vi "Generate LabVIEW FPGA Code for Exponentially Weighted Moving Average Filter.vi"() -> ()   [LabVIEW 2023]
doc: "Demonstrates how to use the Digital Filter Design VIs to design, analyze, and generate LabVIEW FPGA code from a fixed-point, exponentially weighted moving average filter.\n\nComplete the following steps to use this VI.\n1) Specify a valid <B>Destination Folder</B> for code generation.\n2) Specify a <B>Filter Name</B> for code generation.\n3) Specify the number of channels that you want the filter to process in the <B># Channels</B> input.\n4) Run the VI. The <B>Maximum Input Fs@40 MHz FPGA Clock</B> output returns a value that indicates the processing power of the generated filter block."
uses:
  <vilib>/addons/Digital Filter Design/FXPModel.llb/DFD FXP Quantize Coef (Easy).vi
  <vilib>/addons/Digital Filter Design/Analysis.llb/DFD Plot Freq Response (Linear-Spaced).vi
  <vilib>/addons/Digital Filter Design/CodeGen.llb/DFD FXP LabVIEW FPGA Code Generator.vi
  <vilib>/addons/Digital Filter Design/NI_DigFilterLicensed.lvlib
panel:
  out "Magnitude Response":cluster{"f0":dbl, "df":dbl, "values":dbl[]}[](graph)
  in  "Coefficients b/v Word Length":i16=16
  in  "Coefficients a/k Word Length":i16=16
  in  "Sampling Frequency [Hz]":dbl=1000.0 format="%0.2f"
  in  "Time Constant [s]":dbl=0.1 format="%.2f"
  in  "Gain Settings":T1={"gain processing"=1, "gain word length"=16} {"gain processing" items=["On Target", "On Host"]}
  out "Maximum Input Fs@40 MHz FPGA Clock":dbl format="%#_5p Hz"
  out "lvproj Path":path
  in  "Open Project?":bool=TRUE
  in  "Filter Name":string
  in  "# Channels":i32=1
  in  "Destination Folder":path
  in  "Output Word Length":i16=16
  in  "Input Word Length":i16=16
  out "Error Message":string
  # "Select Help>>Show Context Help and move the cursor over the VI icon for more information."
  # "Filter Settings"
  # "Modeling Settings"
  # "Code Generation Settings"
  # "Code Generation Feedback"
  # "Quantization Settings"
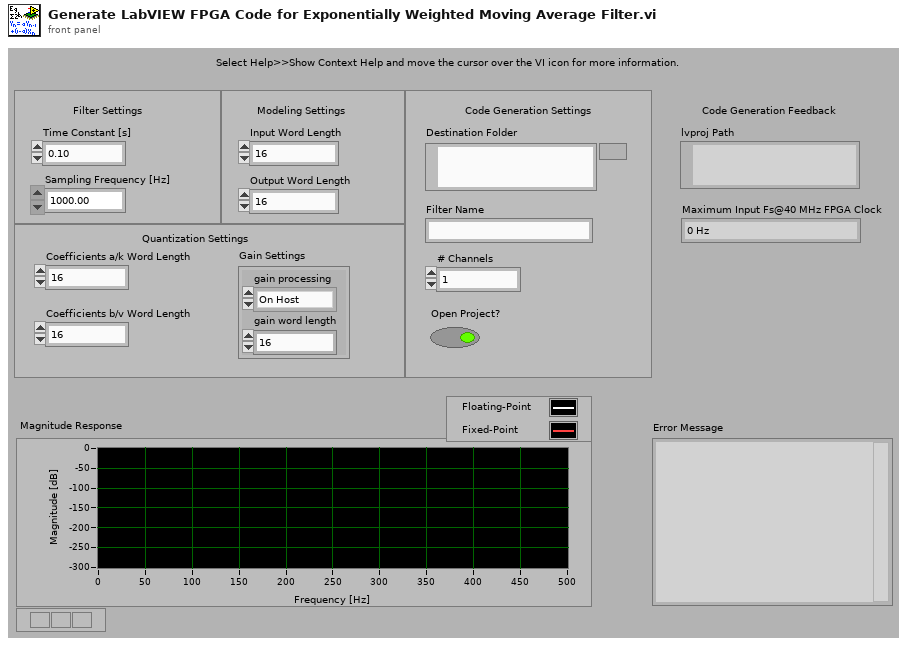
[diagram p1: front panel]
types:
  T1 = cluster{"gain processing":u16, "gain word length":i16}
  T2 = typedef "NI_DigFilterLicensed.lvlib/DFD Filter Obj.ctl" = cluster{"mSRate_Fs":dbl, "mSRate_Version":string, "mSRate_Comments":string, "mSRate_OrgCoef":T3, "mSRate_CurCoef":T3, "mSRate_Quantized?":bool, "mSRate_QCoef":T3, "mSRate_QSettings":T5[], "mSRate_Order":i32, "mSRate_Scaling":cluster{"mSRate_ScaleByPowerOf2?":bool, "mSRate_ScaleType":T7}}
  T3 = typedef "NI_DigFilterLicensed.lvlib/DFD Filter Coef.ctl" = cluster{"type":T4, "gain":dbl, "coef a (k)":dbl[], "coef b (v)":dbl[]}
  T4 = typedef "NI_DigFilterLicensed.lvlib/DFD Filter Structure Type Selector.ctl" = enum16{"Undefined", "FIR Direct Form", "FIR Direct Form Transposed", "FIR Symmetric", "FIR Antisymmetric", "IIR Direct Form I", "IIR Direct Form I Transposed", "IIR Direct Form II", "IIR Direct Form II Transposed", "IIR Cascaded Second Order Sections Form I", "IIR Cascaded Second Order Sections Form I Transposed", "IIR Cascaded Second Order Sections Form II", "IIR Cascaded Second Order Sections Form II Transposed", "Lattice Allpass (basic sections)", "Lattice Allpass (one multiplier sections)", "Lattice Allpass (normalized sections)", "Lattice AR (basic sections)", "Lattice AR (one multiplier sections)", "Lattice AR (normalized sections)", "Lattice MA (minimum phase)", "Lattice MA (maximum phase)", "Lattice ARMA (basic sections)", "Lattice ARMA (one multiplier sections)", "Lattice ARMA (normalized sections)"}
  T5 = typedef "NI_DigFilterLicensed.lvlib/dfd_Internal Quantization Settings.ctl" = cluster{"source":T6, "wl":i16, "iwl":i16, "overflow mode":enum16{"Saturation", "Wrap"}, "rounding mode":enum16{"Nearest", "Truncation"}, "signed?":bool}
  T6 = typedef "NI_DigFilterLicensed.lvlib/dfd_Internal Quantization Srcs.ctl" = u16
  T7 = typedef "NI_DigFilterLicensed.lvlib/DFD Coef Norm Type.ctl" = enum16{"No Norm", "Time Domain 1-Norm", "Time Domain 2-Norm", "Time Domain Inf-Norm"}
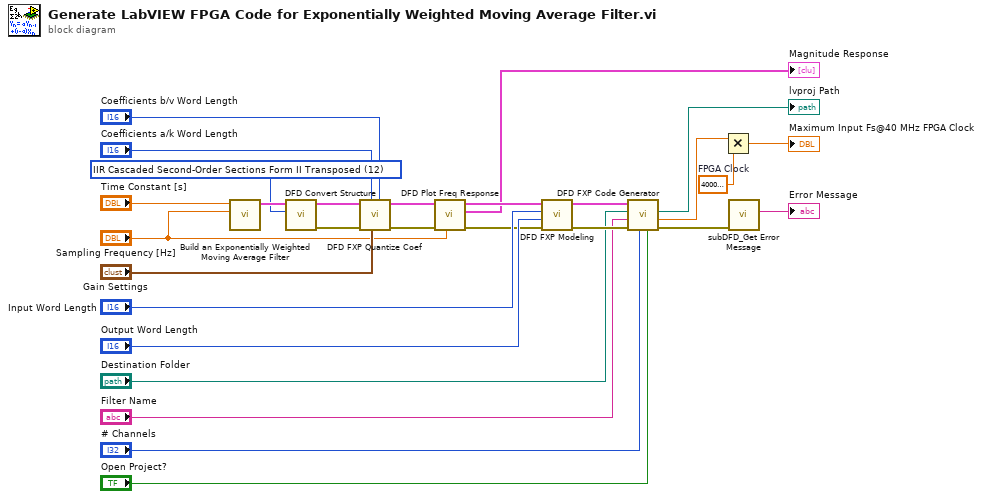
[diagram p0: block diagram]
diagram:
  w8 = u16 12 items=["FIR Direct Form"=1, "FIR Direct Form Transposed"=2, "FIR Symmetric"=3, "FIR Antisymmetric"=4, "IIR Direct Form I"=5, "IIR Direct Form I Transposed"=6, "IIR Direct Form II"=7, "IIR Direct Form II Transposed"=8, "IIR Cascaded Second-Order Sections Form I"=9, "IIR Cascaded Second-Order Sections Form I Transposed"=10, "IIR Cascaded Second-Order Sections Form II"=11, "IIR Cascaded Second-Order Sections Form II Transposed"=12, "Lattice Allpass (basic sections)"=13, "Lattice Allpass (one multiplier sections)"=14, "Lattice Allpass (normalized sections)"=15, "Lattice AR (basic sections)"=16, "Lattice AR (one multiplier sections)"=17, "Lattice AR (normalized sections)"=18, "Lattice MA (minimum phase)"=19, "Lattice MA (maximum phase)"=20, "Lattice ARMA (basic sections)"=21, "Lattice ARMA (one multiplier sections)"=22, "Lattice ARMA (normalized sections)"=23] ("target structure")
  w1 = 40000000.0  # FPGA Clock
  n1 = call "Build an Exponentially Weighted Moving Average Filter.vi"("Sampling Frequency [Hz]"="Sampling Frequency [Hz]", "Time Constant [s]"="Time Constant [s]") -> ("filter out"=w11:T2)  [unwired: 9 out]
  n2 = call <vilib>:"DFD Convert Structure.vi"("target structure"=w8, "filter in"=w11) -> ("error out"=w9:errorcluster, "filter out"=w10:T2)  [unwired: 1 in, 7 out]
  n3 = call-poly <vilib>:"DFD FXP Quantize Coef.vi"("coefficients b/v word length"="Coefficients b/v Word Length", "gain settings"="Gain Settings", "coefficients a/k word length"="Coefficients a/k Word Length", "error in (no error)"=w9, "filter in"=w10) -> ("error out"=w6:errorcluster, "filter out"=w7:T2)  [unwired: 5 out]
  n4 = call-poly <vilib>:"DFD Plot Freq Response.vi"("fs [Hz]"="Sampling Frequency [Hz]", "error in (no error)"=w6, "filter in"=w7) -> ("error out"=w5:errorcluster, "magnitude response"=→"Magnitude Response":cluster{"f0":dbl, "df":dbl, "values":dbl[]}[], "filter out"=w4:T2)  [unwired: 5 in, 1 out]
  n5 = call <vilib>:"DFD FXP Modeling.vi"("error in (no error)"=w5, "output word length"="Output Word Length", "input word length"="Input Word Length", "filter in"=w4) -> ("error out"=w24:errorcluster, "filter out"=w25:T2)  [unwired: 3 in, 3 out]
  n6 = call-poly <vilib>:"DFD FXP Code Generator.vi"("open project? (F)"="Open Project?", "# channels"="# Channels", "error in (no error)"=w24, "filter name"="Filter Name", "destination folder"="Destination Folder", "filter in"=w25) -> ("error out"=w16:errorcluster, "sampling frequency/FPGA clock"=w18:dbl, "lvproj path"=→"lvproj Path":path)  [unwired: 1 in, 2 out]
  n7 = Multiply(x=w18, y=w1) -> (x*y=→"Maximum Input Fs@40 MHz FPGA Clock":dbl)
  n8 = call <vilib>:"subDFD_Get Error Message.vi"("error in (no error)"=w16) -> ("Error Message"=→"Error Message":string)  [unwired: 10 out]
